vi "Get Time.vi"(8 "error IO":errorcluster, 11 "VISA resource name":refnum<visa-resource-name>) -> (0 "error Out":errorcluster, 2 "Time String":string, 3 "VISA resource Out":refnum<visa-resource-name>)   [LabVIEW 2020, in "Associated Research 78XX Series.lvlib"]
uses:
  <instrlib>/Associated Research 78XX Series/Associated Research 78XX Series.lvlib
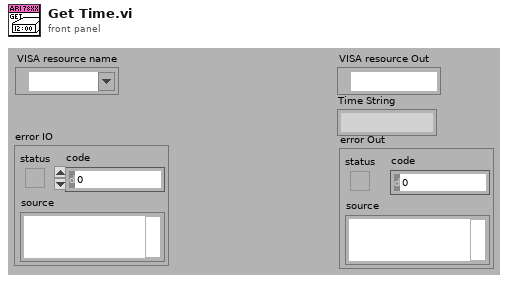
[diagram p1: front panel]
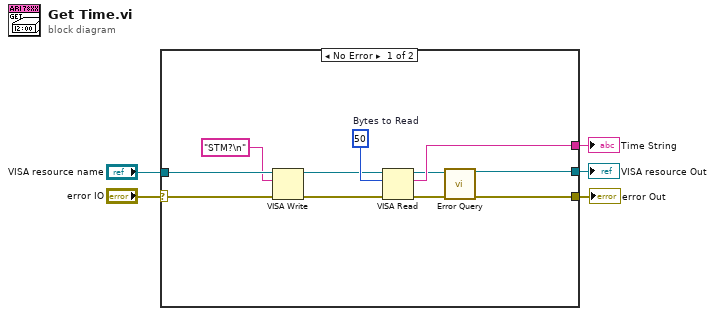
[diagram p0: block diagram]
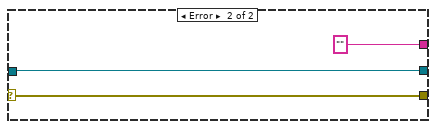
[diagram p2: hidden frame]
diagram:
  n1 = case shown="No Error" "error IO" {
    selector: "error IO" -> [w16 w19]
    tunnel: [w13 w19] -> w1
    tunnel: [w14 w18] -> w3
    tunnel: "VISA resource name" -> [w15 w18]
    tunnel: [w12 "" ("read buffer")] -> w2
    frame No Error {
      w10 = u32 50  # Bytes to Read
      n2 = VISA Write(VISA resource name=w15, write buffer="STM?\n" ("Command to Send (empty)"), error in (no error)=w16) -> (VISA resource name out=w7:refnum<visa-resource-name>, error out=w6:errorcluster)  [unwired: 1 out]
      n3 = VISA Read(VISA resource name=w7, byte count=w10, error in (no error)=w6) -> (VISA resource name out=w9:refnum<visa-resource-name>, read buffer=w12:string, error out=w8:errorcluster)  [unwired: 1 out]
      n4 = call <instrlib>:"Error Query.vi"("VISA resource name"=w9, "error in (no error)"=w8) -> ("VISA resource name out"=w14:refnum<visa-resource-name>, "error out"=w13:errorcluster)  [unwired: 10 in, 2 out]
    }
    frame Error {
    }
  }
  "VISA resource Out" <- w3
  "Time String" <- w2
  "error Out" <- w1
